vi "TEST.vi"   [LabVIEW 2011]
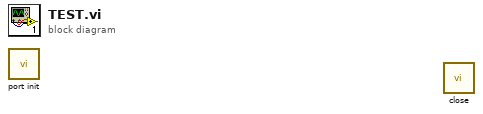
[diagram p0: block diagram]
diagram:
  n1 = call <instrlib>:"port init.vi"() -> ()  [unwired: 4 in, 2 out]
  n2 = call <instrlib>:"close.vi"() -> ()  [unwired: 5 in, 1 out]
